vi "Classify Tips.vi"(8 "error in (no error)":errorcluster, 9 "Image Array":T1[](array[typedef]), 10 "Classifier File":path, 11 "Tips":T2[](array[typedef]) {"ROI Descriptor"."Contours"."Type" items=["No Selection", "Point", "Line", "Rectangle", "Oval", "Polygon", "Freehand Region", "Annulus", "Unused2", "Unused3", "Broken Line", "Freehand Line", "Rotated Rectangle"]; "Point"."Y" format="%.2f"; "Point"."X" format="%.2f"}) -> (0 "error out":errorcluster, 3 "Classified Tips":T2[](array[typedef]) {"ROI Descriptor"."Contours"."Type" items=["No Selection", "Point", "Line", "Rectangle", "Oval", "Polygon", "Freehand Region", "Annulus", "Unused2", "Unused3", "Broken Line", "Freehand Line", "Rotated Rectangle"]; "Point"."Y" format="%.2f"; "Point"."X" format="%.2f"})   [LabVIEW 2013]
uses:
  Controls/Tip.ctl
  <vilib>/vision/Image Controls.llb/IMAQ Image.ctl
  <vilib>/vision/NI_Vision_Development_Module.lvlib
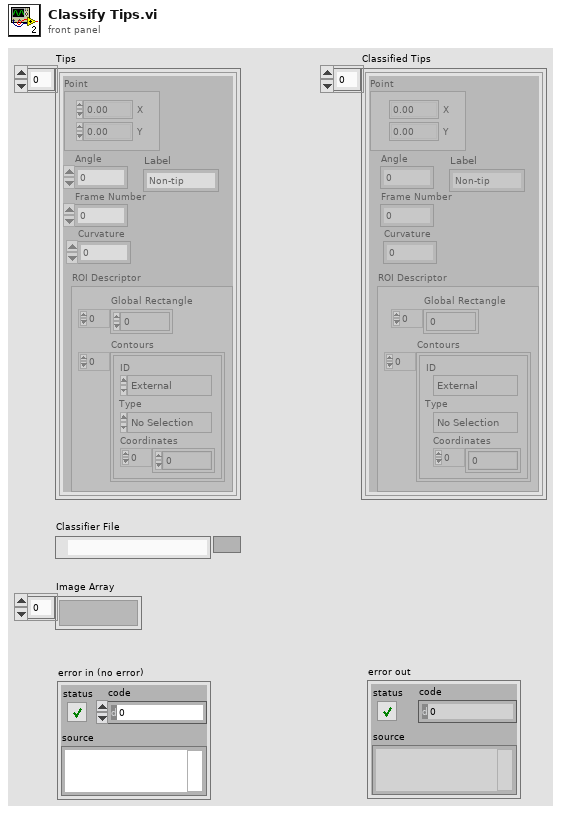
[diagram p1: front panel]
types:
  T1 = typedef "IMAQ Image.ctl" = refnum<image>
  T2 = typedef "Tip.ctl" = cluster{"Point":T3, "Angle":dbl, "Frame Number":i32, "ROI Descriptor":T4, "Curvature":dbl, "Label":string}
  T3 = typedef "IMAQ Point" = cluster{"X":sgl, "Y":sgl}
  T4 = typedef "ROI Descriptor" = cluster{"Global Rectangle":i32[], "Contours":cluster{"ID":enum32{"External", "Internal"}, "Type":u32, "Coordinates":i32[]}[]}
  T5 = typedef "IMAQ Classifier Session.ctl" = refnum<k1>
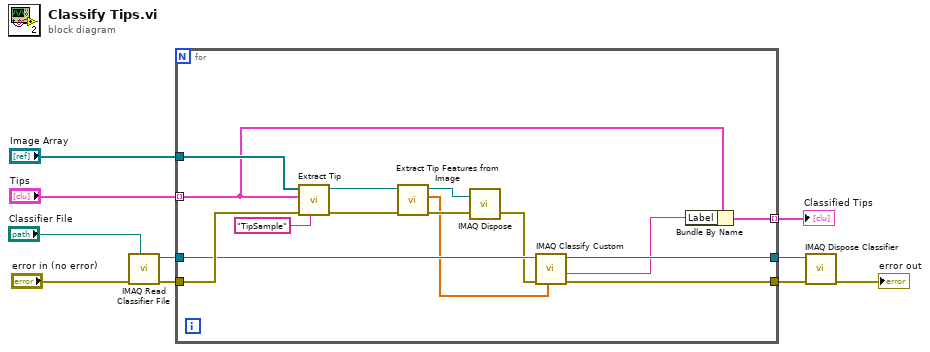
[diagram p0: block diagram]
diagram:
  n1 = call "IMAQ Read Classifier File"("File Path"="Classifier File", "error in (no error)"="error in (no error)") -> ("error out"=w6:errorcluster, "Classifier Session"=w7:T5)  [unwired: 5 in, 3 out]
  n2 = for {
    tunnel: w7 -> [w20]
    tunnel: w6 -> [w21]
    tunnel: "Tips" -> [w18] mode=indexing
    tunnel: "Image Array" -> [w25]
    tunnel: [w19] -> w2
    tunnel: [w16] -> w1
    tunnel: [w15] -> w3 mode=indexing
    n3 = call "Extract Tip.vi"("Label"="TipSample", "error in (no error)"=w21, "Tip"=w18, "Image Array"=w25) -> ("error out"=w22:errorcluster, "Tip Image"=w23:T1)  [unwired: 6 in]
    n4 = call "Extract Tip Features from Image.vi"("error in (no error)"=w22, "Image In"=w23) -> ("error out"=w14:errorcluster, "Features"=w13:dbl[], "Image Out"=w12:T1)  [unwired: 7 in]
    n5 = call "IMAQ Dispose"("Image"=w12, "error in (no error)"=w14) -> ("error out"=w11:errorcluster)  [unwired: 4 in]
    n6 = call "IMAQ Classify Custom"("Feature Vector"=w13, "error in (no error)"=w11, "Classifier Session"=w20) -> ("error out"=w16:errorcluster, "Class"=w17:string, "Classifier Session (dup)"=w19:T5)  [unwired: 3 in, 3 out]
    n7 = Bundle By Name(cluster=w18, "Label"=w17) -> (w15:T2)
  }
  "Classified Tips" <- w3
  n8 = call "IMAQ Dispose Classifier"("error in (no error)"=w1, "Classifier Session"=w2) -> ("error out"=→"error out":errorcluster)  [unwired: 9 in]
